vi "RemoveOrGetExt.vi"(9 "Longitud de la cadena":i32, 10 "String in":string, 11 "Extension-T-Nombre-F":bool) -> (3 "String out":string)   [LabVIEW 2017]
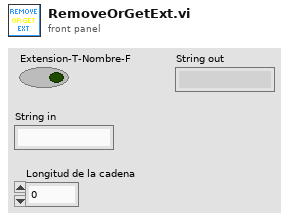
[diagram p1: front panel]
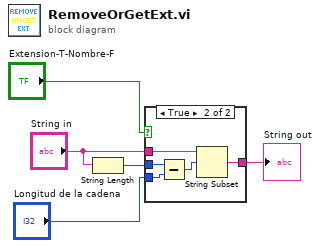
[diagram p0: block diagram]
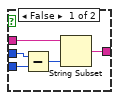
[diagram p2: hidden frame]
diagram:
  n1 = String Length(string="String in") -> (length=w2:i32)
  n2 = case shown="True" "Extension-T-Nombre-F" {
    tunnel: [w7 w15] -> w1
    tunnel: w2 -> [w9 w14]
    tunnel: "String in" -> [w10 w13]
    tunnel: "Longitud de la cadena" -> [w8 w11]
    frame False {
      n3 = Subtract(x=w9, y=w8) -> (x-y=w6:i32)
      n4 = String Subset(string=w10, length (rest)=w6) -> (substring=w7:string)  [unwired: 1 in]
    }
    frame True {
      n5 = Subtract(x=w14, y=w11) -> (x-y=w12:i32)
      n6 = String Subset(string=w13, offset (0)=w12) -> (substring=w15:string)  [unwired: 1 in]
    }
  }
  "String out" <- w1
